vi "MB_TCP_7018_pp.vi"(6 "N":i32, 9 "timeouts":T1={"conn_timeout"=1000, "reconn_timeout"=3000, "N attempt max"=3, "t_reset_TTL"=120000, "write_timeout"=10, "read_timeout"=500, "period"=100} {"t_reset_TTL" min=10 max=240000 step=1; "period" min=10 max=100000 step=1; "read_timeout" min=10 max=60000 step=1; "write_timeout" min=1 max=60000 step=1; "N attempt max" min=1 max=5 step=1; "reconn_timeout" min=10 max=240000 step=1; "conn_timeout" min=10 max=240000}, 10 "write enable":bool=TRUE, 11 "stop":bool) -> (0 "error out":errorcluster, 2 "errors":u32, 3 "Z3":u32)   [LabVIEW 2019]
uses:
  NI_modbus_upd/NI_modbus_upd.lvlib
  NI_modbus_upd1.llb/MB Modbus Command.ctl
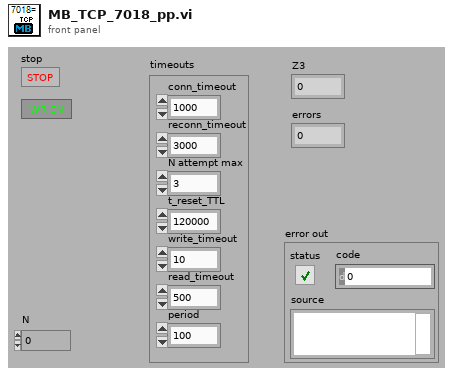
[diagram p1: front panel]
types:
  T1 = cluster{"conn_timeout":i32, "reconn_timeout":u32, "N attempt max":i32, "t_reset_TTL":u32, "write_timeout":i32, "read_timeout":i32, "period":u32}
  T2 = enum16{"Init", "Read", "Read inputs", "Read outputs", "Write", "Write inputs"}
  T3 = enum16{"DI", "DO to write", "DO", "AI", "AO to write", "AO", "DI AI", "DI AO", "DO AI", "DO AO"}
  T4 = enum16{"Start", "Connect", "Write enable", "IP address", "Errors"}
  T5 = cluster{"Transaction ID":u16, "Protocol ID":u16, "Length":u16, "Unit ID":u8}
  T6 = typedef "MB Modbus Command.ctl" = cluster{"Function Code":u8, "Starting Address":u16, "Quantity":u16, "Data":u16[], "Discrete":bool[]}
  T7 = cluster{"Remote IP Address":string, "Remote Port":u16}
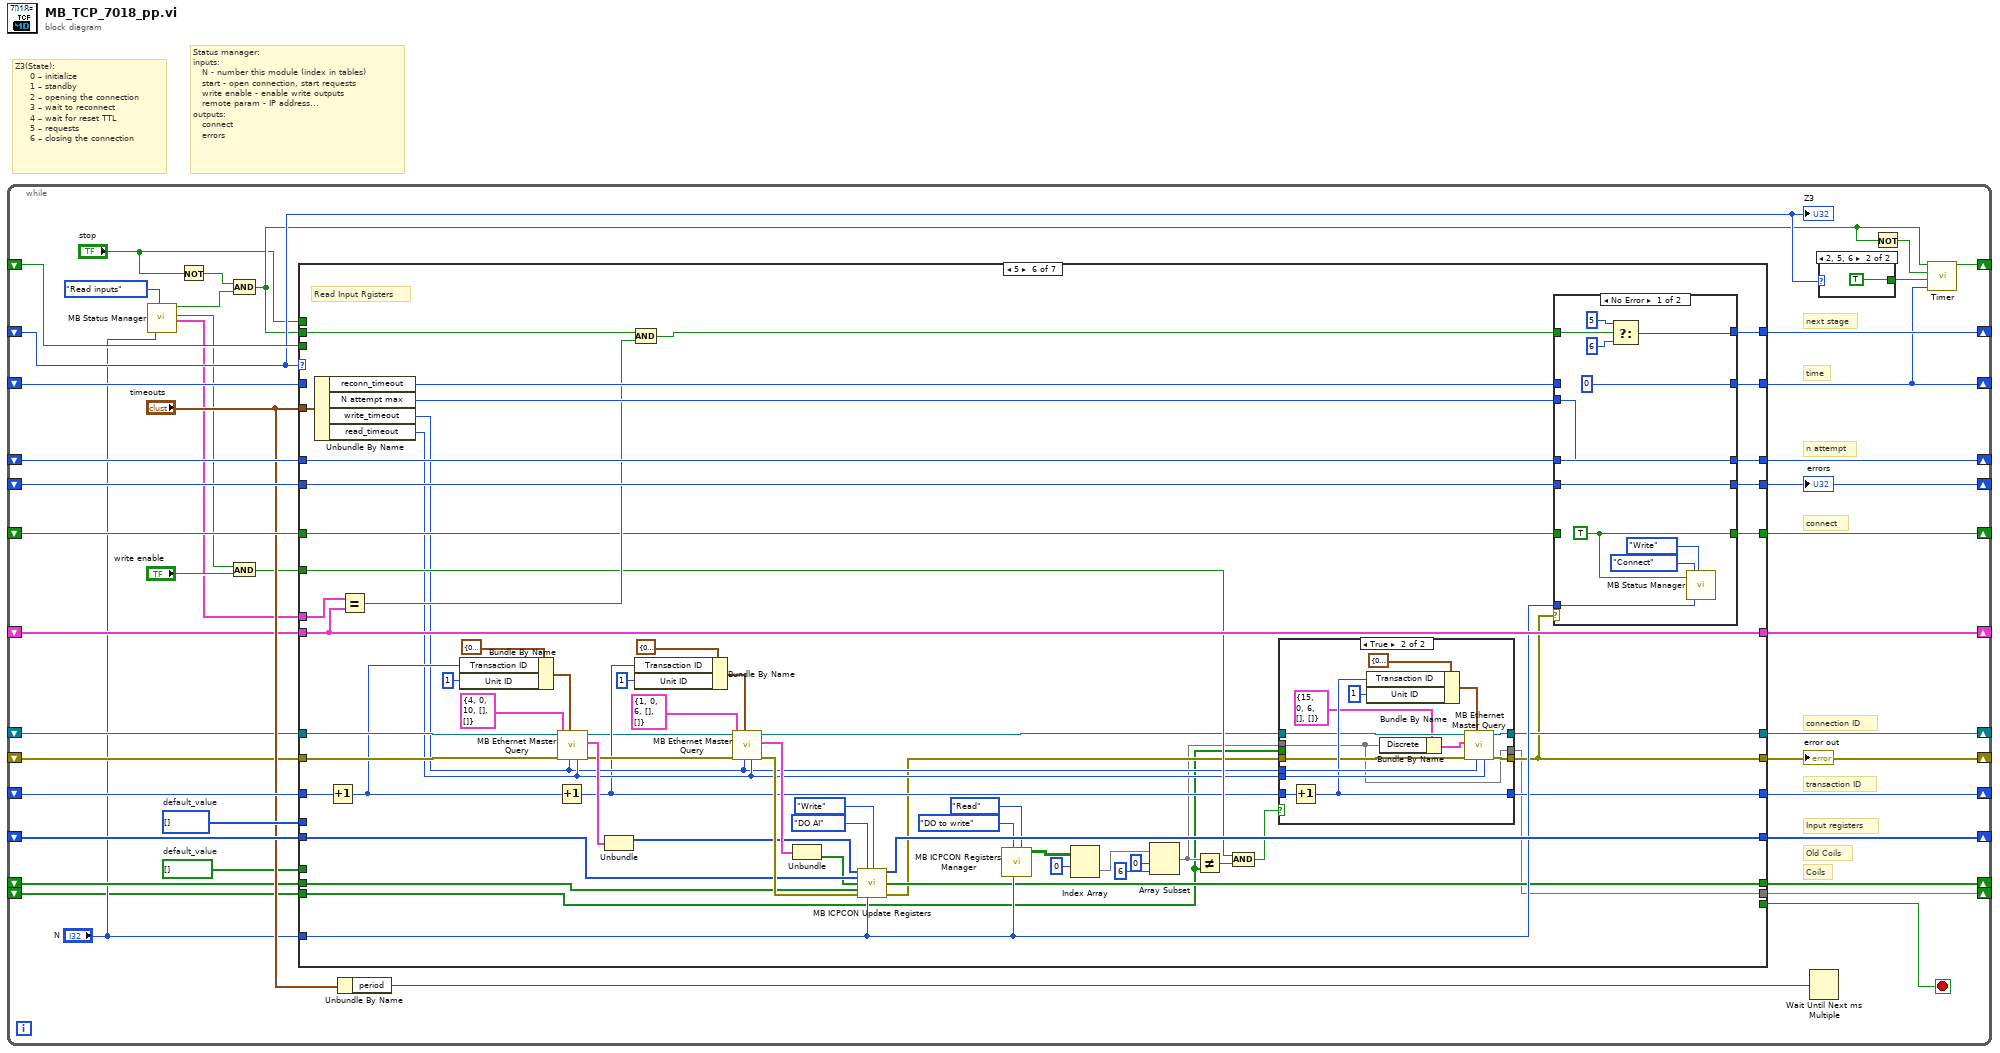
[diagram p0: block diagram]
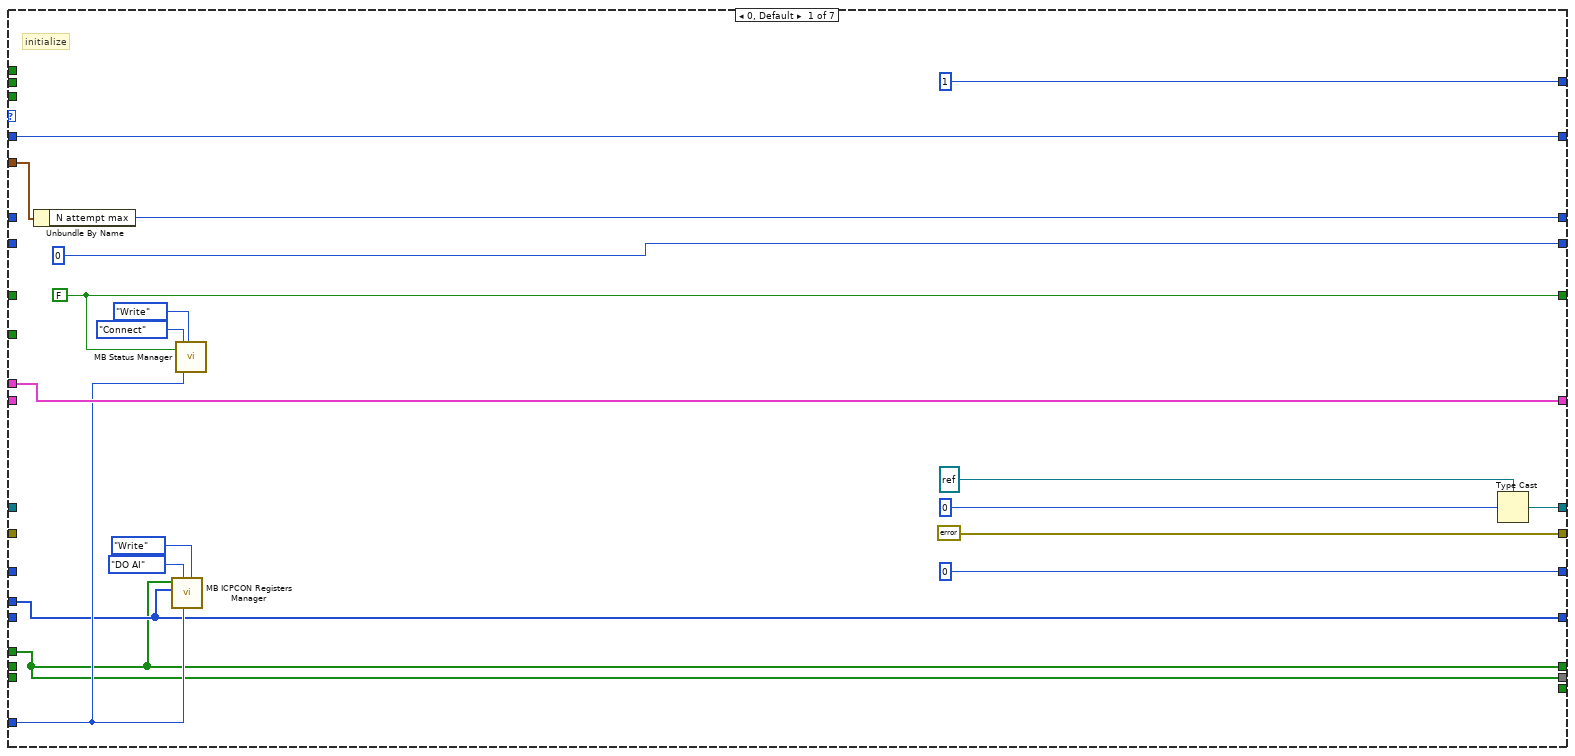
[diagram p2: hidden frame]
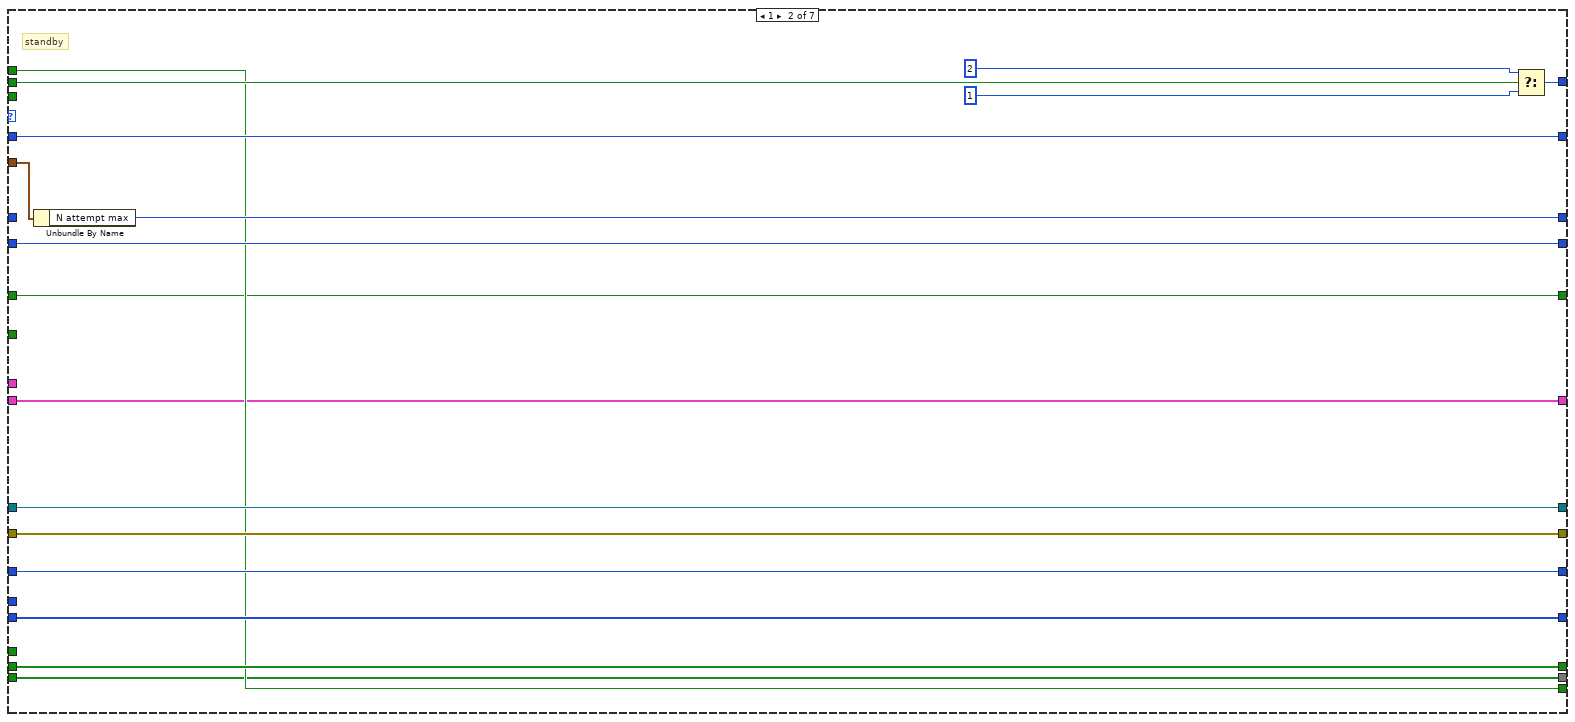
[diagram p3: hidden frame]
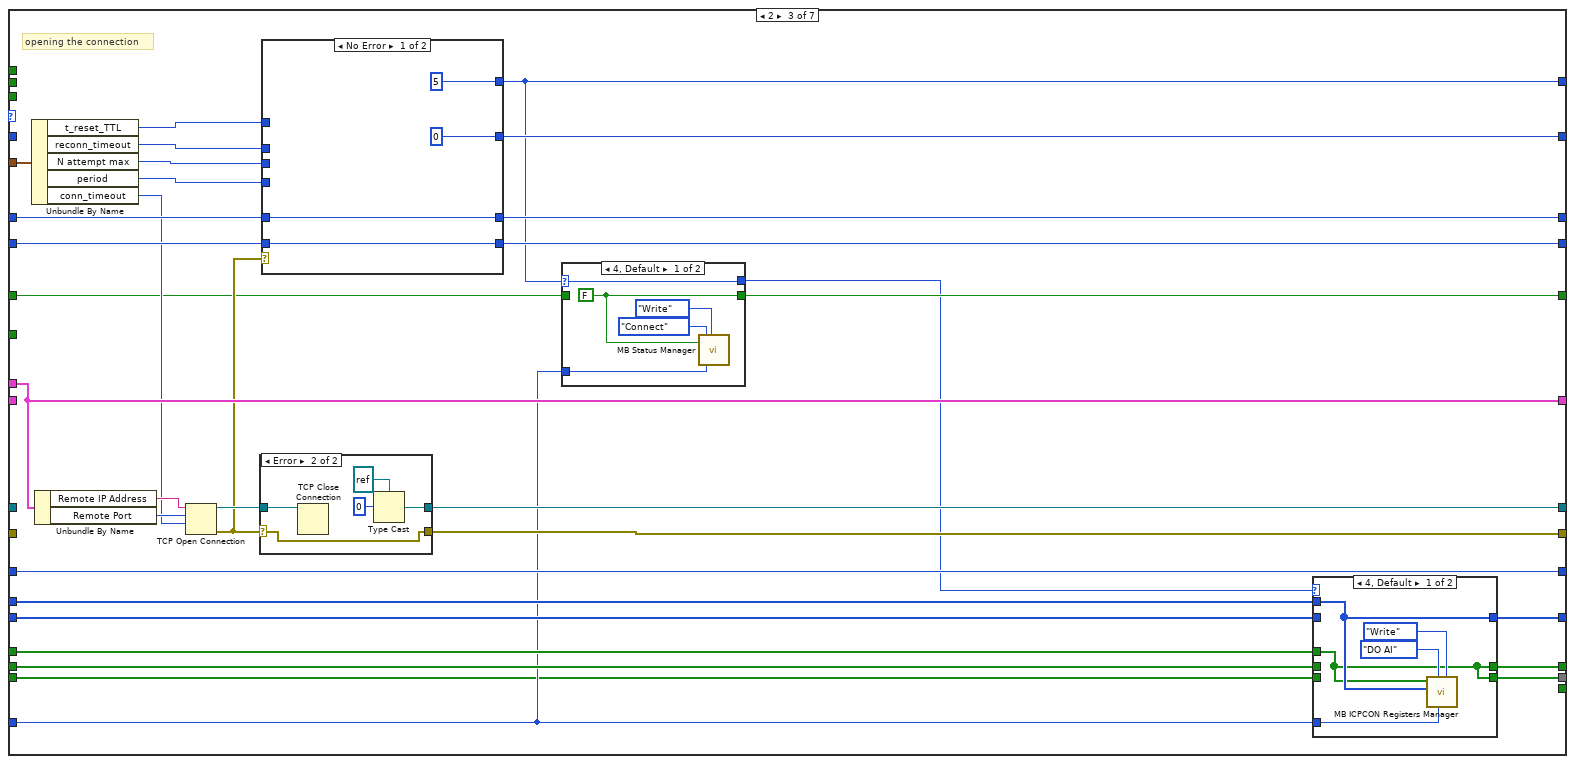
[diagram p4: hidden frame]
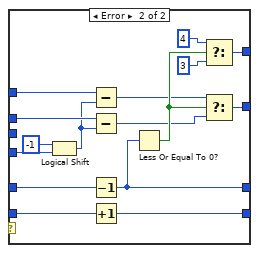
[diagram p8: hidden frame]
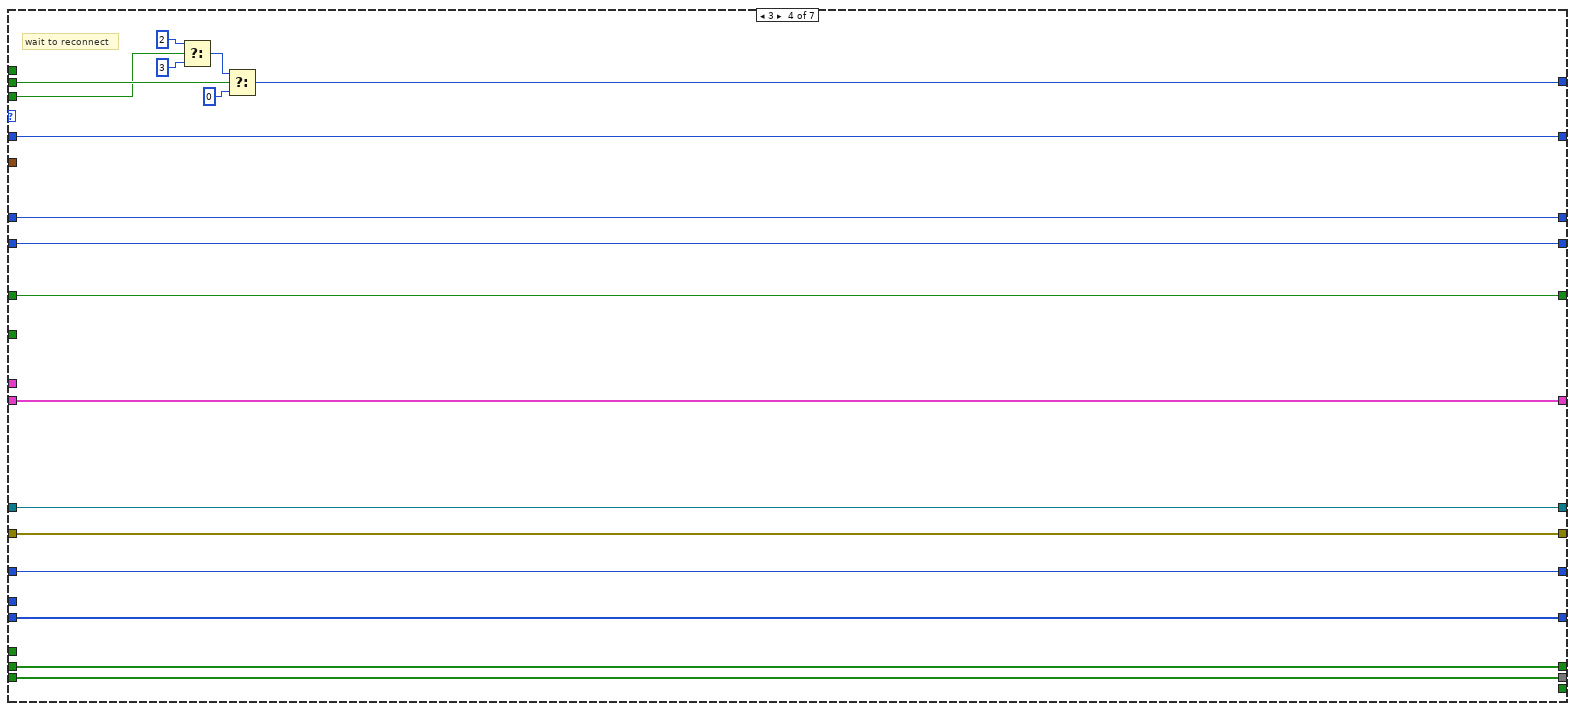
[diagram p9: hidden frame]
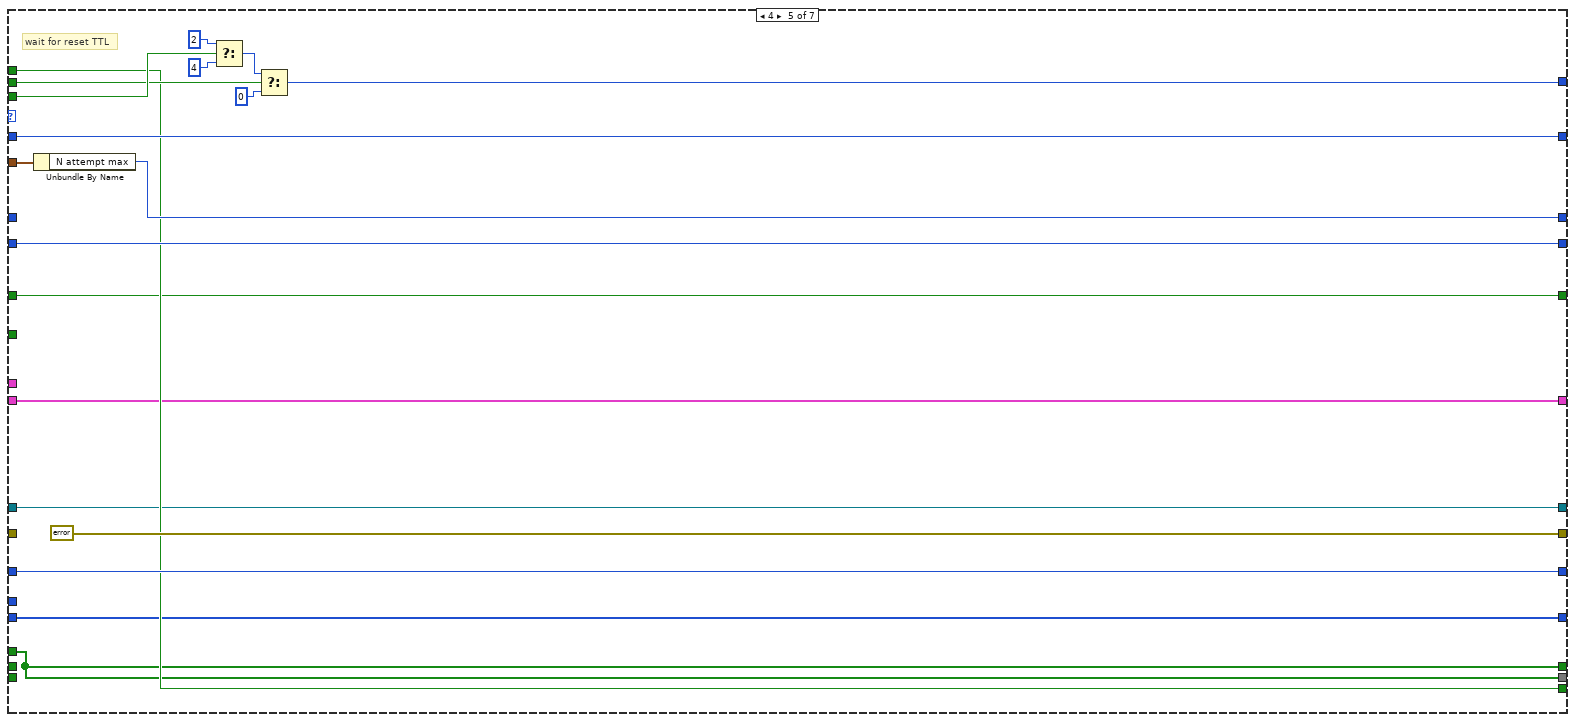
[diagram p10: hidden frame]
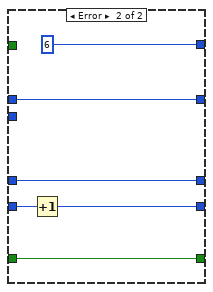
[diagram p12: hidden frame]
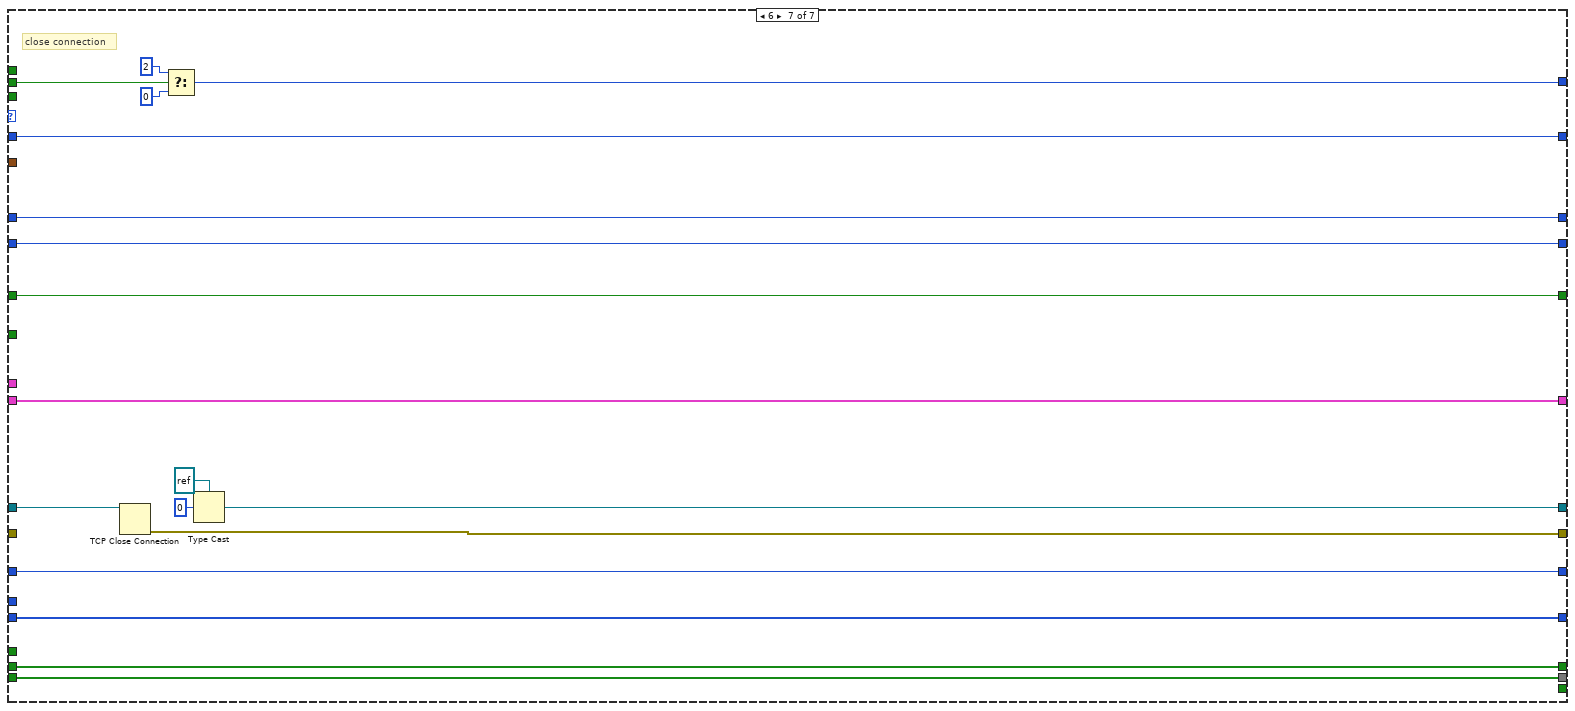
[diagram p13: hidden frame]
diagram:
  # "Status manager:\ninputs:\n   N - number this module (index in tables)\n   start - open connection, start requests\n   write enable - enable write outputs\n   remote param - IP address...\noutputs:\n   connect\n   errors"
  # "Z3(State):\n     0 – initialize \n     1 – standby\n     2 – opening the connection\n     3 – wait to reconnect\n     4 – wait for reset TTL\n     5 – requests\n     6 – closing the connection"
  n1 = while {
    shift-right: [w20] -> _
    shift-left: _ -> [w16]
    shift-right: [w19] -> _
    shift-left: _ -> [w42]
    shift-right: [w41] -> _
    shift-left: _ -> [w39]
    shift-right: [w40] -> _
    shift-left: _ -> [w38]
    shift-right: [w37] -> _
    shift-left: _ -> [w36]
    shift-right: [w35] -> _
    shift-left: _ -> [w21]
    shift-right: [w34] -> _
    shift-left: _ -> [w22]
    shift-right: [w33] -> _
    shift-left: _ -> [w32]
    shift-right: [w31] -> _
    shift-left: _ -> [w30]
    shift-right: [w24] -> _
    shift-left: _ -> [w23]
    shift-right: [w18] -> _
    shift-left: _ -> [w17]
    shift-right: [w9] -> _
    shift-left: _ -> [w8]
    shift-right: [w2] -> _
    shift-left: _ -> [w1]
    stop <- w12 stop-if-true
    w25 = bool[] []  # default_value
    w29 = u16[] []  # default_value
    # "Old Coils"
    # "Coils"
    # "Input registers"
    # "connect"
    # "connection ID"
    # "transaction ID"
    # "n attempt"
    # "time"
    # "next stage"
    n2 = call "MB Status Manager.vi"("N"="N", "Function"=T2."Read inputs") -> ("start"=w6:bool, "write enable"=w5:bool, "Remote Param"=w4:T7)  [unwired: 12 in, 3 out]
    n3 = Not(x="stop") -> (.not. x?=w14:bool)
    n4 = And(x=w14, y=w6) -> (x .and. y?=w15:bool)
    n5 = And(x=w5, y="write enable") -> (x .and. y?=w11:bool)
    n6 = case shown="5" w16 {
      tunnel: [w60 w70 w89 w169 w176 w202 w303] -> w35
      tunnel: [errorcluster {"status"=FALSE, "code"=0, "source"=""} ("error out") w69 w87 w168 errorcluster {"status"=FALSE, "code"=0, "source"=""} ("error out") w201 w304] -> w34
      tunnel: w21 -> [_ w70 _ w169 w176 w243 w300]
      tunnel: w22 -> [_ w69 _ w168 _ w242 _]
      tunnel: [w49 w65 w85 w157 w175 w230 w291] -> w37
      tunnel: w36 -> [_ w65 w86 w157 w175 w231 w291]
      tunnel: w4 -> [w52 _ w92 _ _ w237 _]
      tunnel: [w47 w71 w97 w156 w174 w227 w290] -> w31
      tunnel: w30 -> [_ w71 w98 w156 w174 w196 w290]
      tunnel: w32 -> [_ w79 w111 w171 w190 w252 w305]
      tunnel: [u16 0 ("x") w79 w111 w171 w190 w204 w305] -> w33
      tunnel: [w54 w75 w106 w170 w186 w250 w297] -> w41
      tunnel: w39 -> [_ _ w107 w170 _ w250 w297]
      tunnel: [u32 0 ("N attempt max") w78 w109 w167 w189 w249 w302] -> w40
      tunnel: w38 -> [_ w78 w110 w167 w189 w248 w302]
      tunnel: [w56 w77 w103 w166 w188 w245 w301] -> w19
      tunnel: w42 -> [w56 w77 _ w166 w188 _ w301]
      tunnel: "timeouts" -> [w55 w76 w108 _ w187 w251 _]
      tunnel: w15 -> [_ w67 _ w162 w178 w236 w298]
      tunnel: [u32 1 w72 w83 w158 w181 w244 w292] -> w20
      tunnel: w17 -> [_ _ _ w160 w180 _ _]
      tunnel: w29 -> [w47 _ w96 _ _ _ _]
      tunnel: w25 -> [w44 _ w93 _ w172 _ _]
      tunnel: [w44 w68 w94 w159 w172 w208 w295] -> w24
      tunnel: w23 -> [_ w68 w95 w159 _ w194 w295]
      tunnel: "N" -> [w48 _ w84 _ _ w212 _]
      tunnel: "stop" -> [_ w66 _ _ w177 _ _]
      tunnel: [_ w66 _ _ w177 _ _] -> w12
      tunnel: w11 -> [_ _ _ _ _ w215 _]
      tunnel: [w52 w64 w92 w155 w173 w234 w289] -> w9
      tunnel: w8 -> [_ w64 _ w155 w173 w234 w289]
      tunnel: [w44 w63 w80 w154 w172 w191 w288] -> w2
      tunnel: w1 -> [_ w63 w81 w154 _ w192 w288]
      frame 0, Default {
        w49 = FALSE ("connect")
        # "initialize"
        n7 = Unbundle By Name(w55) -> ("N attempt max"=w54:i32)
        n8 = call "MB ICPCON Registers Manager.vi"("Function"=enum16{"Init", "Read", "Write", "Read All"}."Write", "N"=w48, "Table"=T3."DO AI", "Registers In"=w47, "Discrete in"=w44) -> ()  [unwired: 4 in, 3 out]
        n9 = call "MB Status Manager.vi"("connect in"=w49, "Table"=T4."Connect", "N"=w48, "Function"=T2."Write") -> ()  [unwired: 10 in, 6 out]
        n10 = Type Cast(type=refnum<k5> refnum ("connection ID"), x=u32 0) -> (*(type *) &x=w60:refnum<k5>)
      }
      frame 1 {
        # "standby"
        n11 = Unbundle By Name(w76) -> ("N attempt max"=w75:i32)
        n12 = Select(t=u32 2, s=w67, f=u32 1) -> (s? t:f=w72:u32)
      }
      frame 2 {
        # "opening the connection"
        n13 = Unbundle By Name(w108) -> ("t_reset_TTL"=w102:u32, "reconn_timeout"=w104:u32, "N attempt max"=w105:i32, "period"=w99:u32, "conn_timeout"=w91:i32)
        n14 = Unbundle By Name(w92) -> ("Remote IP Address"=w101:string, "Remote Port"=w100:u16)
        n15 = TCP Open Connection(address=w101, remote port or service name=w100, timeout ms (60000)=w91) -> (connection ID=w90:refnum<k5>, error out=w88:errorcluster)  [unwired: 2 in]
        n16 = case shown="Error" w88 {
          selector: w88 -> [w119 w121]
          tunnel: w90 -> [w120 w124]
          tunnel: [w120 w123] -> w89
          tunnel: [w119 w121] -> w87
          frame No Error {
          }
          frame Error {
            n17 = TCP Close Connection(connection ID=w124) -> ()  [unwired: 2 in, 2 out]
            n18 = Type Cast(type=refnum<k5> refnum ("connection ID"), x=u32 0) -> (*(type *) &x=w123:refnum<k5>)
          }
        }
        n19 = case shown="No Error" w88 {
          tunnel: w110 -> [w137 w153]
          tunnel: [w137 w152] -> w109
          tunnel: w107 -> [w136 w151]
          tunnel: [w136 w150] -> w106
          tunnel: w105 -> [_ _]
          tunnel: [u32 5 w147] -> w83
          tunnel: w104 -> [_ w146]
          tunnel: [u32 0 w145] -> w103
          tunnel: w102 -> [_ w142]
          tunnel: w99 -> [_ w140]
          frame No Error {
          }
          frame Error {
            n20 = Logical Shift(y=i16 -1, x=w140) -> (x << y=w138:u32)
            n21 = Subtract(x=w142, y=w138) -> (x-y=w141:u32)
            n22 = Subtract(x=w146, y=w138) -> (x-y=w143:u32)
            n23 = Decrement(x=w151) -> (x-1=w150:i32)
            n24 = Increment(x=w153) -> (x+1=w152:u32)
            n25 = Less Or Equal To 0?(x=w150) -> (x <= 0?=w144:bool)
            n26 = Select(t=u32 4, s=w144, f=u32 3) -> (s? t:f=w147:u32)
            n27 = Select(t=w141, s=w144, f=w143) -> (s? t:f=w145:u32)
          }
        }
        n28 = case shown="4, Default" w83 {
          selector: w83 -> [w113 w117]
          tunnel: w84 -> [w114 _]
          tunnel: [w115 w118] -> w85
          tunnel: w86 -> [_ w118]
          tunnel: [w113 w117] -> w82
          frame 4, Default {
            w115 = FALSE ("f")
            n29 = call "MB Status Manager.vi"("connect in"=w115, "Table"=T4."Connect", "N"=w114, "Function"=T2."Write") -> ()  [unwired: 10 in, 6 out]
          }
          frame 3, 5 {
          }
        }
        n30 = case shown="4, Default" w82 {
          tunnel: w84 -> [w129 _]
          tunnel: [w127 w133] -> w97
          tunnel: w98 -> [_ w133]
          tunnel: w96 -> [w127 _]
          tunnel: w95 -> [_ w132]
          tunnel: [w126 w132] -> w94
          tunnel: w93 -> [w126 _]
          tunnel: w81 -> [_ w131]
          tunnel: [w126 w131] -> w80
          frame 4, Default {
            n31 = call "MB ICPCON Registers Manager.vi"("Function"=enum16{"Init", "Read", "Write", "Read All"}."Write", "N"=w129, "Table"=T3."DO AI", "Registers In"=w127, "Discrete in"=w126) -> ()  [unwired: 4 in, 3 out]
          }
          frame 3, 5 {
          }
        }
      }
      frame 3 {
        # "wait to reconnect"
        n32 = Select(t=u32 2, s=w160, f=u32 3) -> (s? t:f=w161:u32)
        n33 = Select(t=w161, s=w162, f=u32 0) -> (s? t:f=w158:u32)
      }
      frame 4 {
        # "wait for reset TTL"
        n34 = Unbundle By Name(w187) -> ("N attempt max"=w186:i32)
        n35 = Select(t=u32 2, s=w180, f=u32 4) -> (s? t:f=w182:u32)
        n36 = Select(t=w182, s=w178, f=u32 0) -> (s? t:f=w181:u32)
      }
      frame 5 {
        # "Read Input Rgisters"
        n37 = Unbundle By Name(w251) -> ("reconn_timeout"=w246:u32, "N attempt max"=w247:i32, "write_timeout"=w206:i32, "read_timeout"=w207:i32)
        n38 = Increment(x=w252) -> (x+1=w223:u16)
        n39 = Equal?(x=w237, y=w234) -> (x = y?=w233:bool)
        n40 = Bundle By Name(cluster=T5 {"Transaction ID"=0, "Protocol ID"=0, "Length"=0, "Unit ID"=0} ("MBAP Header"), "Transaction ID"=w223, "Unit ID"=u8 1) -> (w238:T5)
        n41 = Increment(x=w223) -> (x+1=w205:u16)
        n42 = call "MB Ethernet Master Query.vi"("Read Timeout"=w207, "Write Timeout"=w206, "MBAP Header"=w238, "error in (no error)"=w242, "Modbus Command"=T6 {"Function Code"=4, "Starting Address"=0, "Quantity"=10, "Data"=[], "Discrete"=[]}, "TCP Connection Refnum in"=w243) -> ("error out"=w221:errorcluster, "Registers"=w241:cluster{"Registers":u16[], "Discrete":bool[]}, "TCP Connection Refnum (dup)"=w200:refnum<k5>)  [unwired: 2 in, 1 out]
        n43 = Unbundle(w241) -> ("Registers"=w197:u16[])  [unwired: 1 out]
        n44 = And(x=w236, y=w233) -> (x .and. y?=w235:bool)
        n45 = Bundle By Name(cluster=T5 {"Transaction ID"=0, "Protocol ID"=0, "Length"=0, "Unit ID"=0} ("MBAP Header"), "Transaction ID"=w205, "Unit ID"=u8 1) -> (w226:T5)
        n46 = call "MB Ethernet Master Query.vi"("Read Timeout"=w207, "Write Timeout"=w206, "MBAP Header"=w226, "error in (no error)"=w221, "Modbus Command"=T6 {"Function Code"=1, "Starting Address"=0, "Quantity"=6, "Data"=[], "Discrete"=[]} ("MODBUS Command"), "TCP Connection Refnum in"=w200) -> ("error out"=w220:errorcluster, "Registers"=w219:cluster{"Registers":u16[], "Discrete":bool[]}, "TCP Connection Refnum (dup)"=w199:refnum<k5>)  [unwired: 2 in, 1 out]
        n47 = Unbundle(w219) -> ("Discrete"=w195:bool[])  [unwired: 1 out]
        n48 = call "MB ICPCON Update Registers.vi"("Registers In"=w197, "Table"=T3."DO AI", "Function"=enum16{"Init", "Read", "Write", "Read All"}."Write", "Default Registers In"=w196, "Discrete in"=w195, "Default Discrete in"=w194, "error in (no error)"=w220, "N"=w212) -> ("Registers"=w227:u16[], "Discretes"=w208:bool[], "error out"=w198:errorcluster)  [unwired: 5 in]
        n49 = call "MB ICPCON Registers Manager.vi"("Function"=enum16{"Init", "Read", "Write", "Read All"}."Read", "N"=w212, "Table"=T3."DO to write") -> ("Discretes"=w211:bool[][])  [unwired: 6 in, 2 out]
        n50 = Index Array(array=w211, index (row)=0) -> (element=w209:bool[])  [unwired: 1 in]
        n51 = Array Subset(array=w209, index=0, length=6) -> (w193:bool[])
        n52 = Not Equal?(x=w193, y=w192) -> (x != y?=w218:bool)
        n53 = And(x=w215, y=w218) -> (x .and. y?=w203:bool)
        n54 = case shown="True" w203 {
          tunnel: w207 -> [_ w268]
          tunnel: w206 -> [_ w267]
          tunnel: w205 -> [w255 w266]
          tunnel: [w255 w265] -> w204
          tunnel: w198 -> [w254 w263]
          tunnel: [w254 w262] -> w201
          tunnel: w199 -> [w256 w261]
          tunnel: [w256 w260] -> w202
          tunnel: w193 -> [_ w257]
          tunnel: w192 -> [w253 _]
          tunnel: [w253 w257] -> w191
          frame False {
          }
          frame True {
            n55 = Increment(x=w266) -> (x+1=w265:u16)
            n56 = Bundle By Name(cluster=T5 {"Transaction ID"=0, "Protocol ID"=0, "Length"=0, "Unit ID"=0} ("MBAP Header"), "Transaction ID"=w265, "Unit ID"=u8 1) -> (w269:T5)
            n57 = Bundle By Name(cluster=T6 {"Function Code"=15, "Starting Address"=0, "Quantity"=6, "Data"=[], "Discrete"=[]} ("MODBUS Command"), "Discrete"=w257) -> (w258:T6)
            n58 = call "MB Ethernet Master Query.vi"("Read Timeout"=w268, "Write Timeout"=w267, "MBAP Header"=w269, "error in (no error)"=w263, "Modbus Command"=w258, "TCP Connection Refnum in"=w261) -> ("error out"=w262:errorcluster, "TCP Connection Refnum (dup)"=w260:refnum<k5>)  [unwired: 2 in, 2 out]
          }
        }
        n59 = case shown="No Error" w201 {
          tunnel: w248 -> [w275 w287]
          tunnel: [w275 w286] -> w249
          tunnel: [w277 u32 6] -> w244
          tunnel: w250 -> [_ w284]
          tunnel: w247 -> [w281 _]
          tunnel: [w281 w284] -> _
          tunnel: w246 -> [_ w283]
          tunnel: [u32 0 w283] -> w245
          tunnel: w235 -> [w276 _]
          tunnel: w231 -> [_ w282]
          tunnel: [w273 w282] -> w230
          tunnel: w212 -> [w272 _]
          frame No Error {
            w273 = TRUE ("f")
            n60 = Select(t=u32 5, s=w276, f=u32 6) -> (s? t:f=w277:u32)
            n61 = call "MB Status Manager.vi"("connect in"=w273, "Table"=T4."Connect", "N"=w272, "Function"=T2."Write") -> ()  [unwired: 10 in, 6 out]
          }
          frame Error {
            n62 = Increment(x=w287) -> (x+1=w286:u32)
          }
        }
      }
      frame 6 {
        # "close connection"
        n63 = TCP Close Connection(connection ID=w300) -> (error out=w304:errorcluster)  [unwired: 2 in, 1 out]
        n64 = Select(t=u32 2, s=w298, f=u32 0) -> (s? t:f=w292:u32)
        n65 = Type Cast(type=refnum<k5> refnum ("connection ID"), x=u32 0) -> (*(type *) &x=w303:refnum<k5>)
      }
    }
    "error out" <- w34
    "errors" <- w40
    n66 = Unbundle By Name("timeouts") -> ("period"=w27:u32)
    n67 = Wait Until Next ms Multiple(millisecond multiple=w27) -> ()  [unwired: 1 out]
    n68 = case shown="2, 5, 6" w16 {
      tunnel: [_ TRUE] -> w26
      frame 0, Default {
      }
      frame 2, 5, 6 {
      }
    }
    n69 = Not(x=w15) -> (.not. x?=w43:bool)
    n70 = call "Timer.vi"("ms"=w19, "Load (F)"=w26, "Reset (F)"=w43, "Start (T)"=w15) -> ("End"=w18:bool)  [unwired: 5 in, 1 out]
    "Z3" <- w16
  }
